vi "Test 1 Move Into 7.vi"(8 "error in (no error)":errorcluster, 11 "Test Case In":refnum<class "Day X Test.lvclass">) -> (0 "error out":errorcluster, 3 "Test Case Out":refnum<class "Day X Test.lvclass">)   [LabVIEW 2020, in "Day X Test.lvclass"]
uses:
  Day X Test.lvclass
  C:/Program Files (x86)/National Instruments/LabVIEW 2020/vi.lib/Astemes/LUnit/Test Case.lvclass
  Map/Position.ctl
  <vilib>/Astemes/LUnit/Test Case.lvclass/Test Case.ctl
  4993e8ee-a06a-463a-9684-69129f64d5ce.vi
  <vilib>/Astemes/LUnit/Append Pass Result.vi
  <vilib>/Astemes/LUnit/Append Fail Result.vi
  <vilib>/Astemes/LUnit/Describe Comparison.vi
  <vilib>/Astemes/LUnit/Compare Variants.vi
  <vilib>/Astemes/LUnit/Variant to string.vi
  <vilib>/Utility/Data Type/Get Type Information.vi
  <vilib>/Utility/LVClass/Get LV Class Name.vi
  Map/Map.lvclass
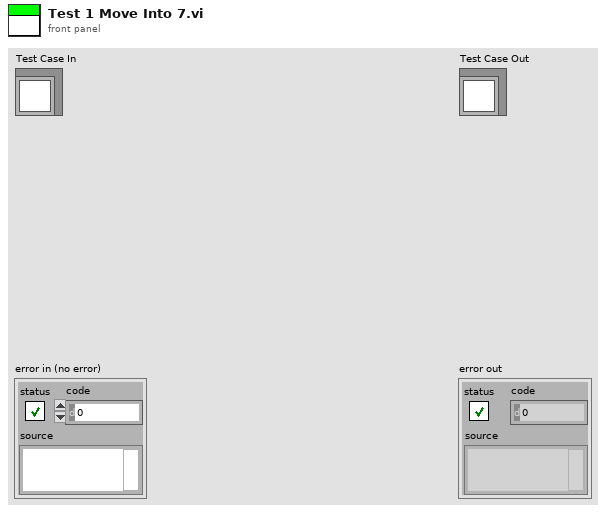
[diagram p1: front panel]
types:
  T1 = typedef "Map.lvclass/Position.ctl" = cluster{"Row":u64, "Col":u64, "Next Move":enum16{"North", "East", "South", "West", "Halt"}}
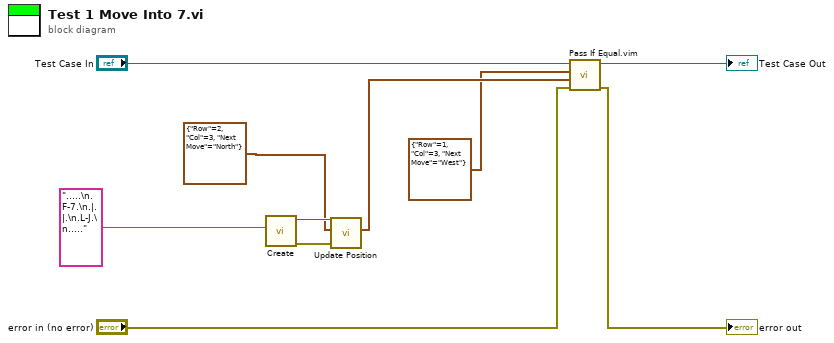
[diagram p0: block diagram]
diagram:
  n1 = call "Create.vi"("Input"=".....\n.F-7.\n.|.|.\n.L-J.\n.....") -> ("error out"=w4:errorcluster, "Map"=w5:refnum<class "Map.lvclass">)  [unwired: 9 in]
  n2 = call "Update Position.vi"("error in (no error)"=w4, "Current"=T1 {"Row"=2, "Col"=3, "Next Move"=enum."North"}, "Map In"=w5) -> ("Next"=w2:T1)  [unwired: 6 in, 2 out]
  n3 = call "Pass If Equal.vim"("error in (no error)"="error in (no error)", "Actual"=w2, "Expected"=T1 {"Row"=1, "Col"=3, "Next Move"=enum."West"}, "LUnit Test Case In"="Test Case In") -> ("error out"=→"error out":errorcluster, "LUnit Test Case Out"=→"Test Case Out":refnum<class "Day X Test.lvclass">)  [unwired: 6 in]
